vi "Create Config File Header.vi"(8 "error in (no error)":errorcluster, 11 "file path":path) -> (0 "error out":errorcluster, 3 "new file path":path)   [LabVIEW 2018, in "Config_Read_SPI.lvclass"]
uses:
  Config_Read_SPI.lvclass
  <vilib>/Utility/file.llb/Write Delimited Spreadsheet (string).vi
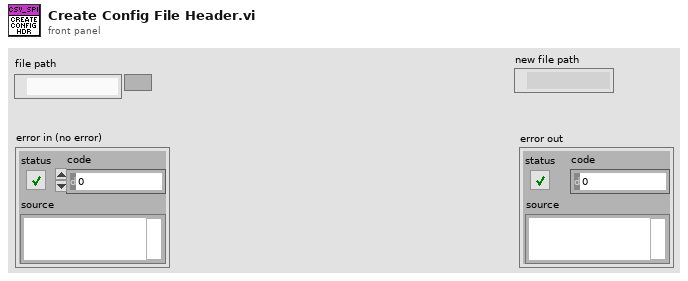
[diagram p1: front panel]
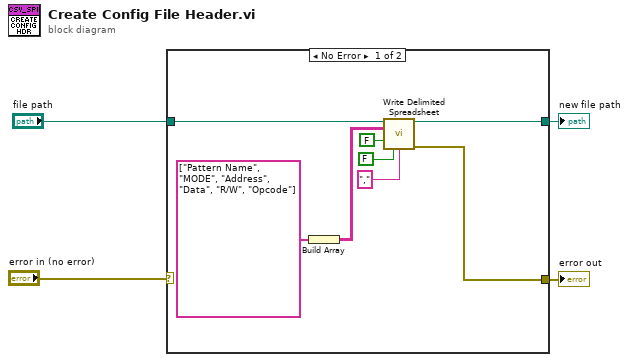
[diagram p0: block diagram]
diagram:
  n1 = case shown="No Error" "error in (no error)" {
    selector: "error in (no error)" -> [_ w13]
    tunnel: "file path" -> [w10 w14]
    tunnel: [w9 w13] -> w1
    tunnel: [w8 w14] -> w2
    frame No Error {
      n2 = Build Array(string[] ["Pattern Name", "MODE", "Address", "Data", "R/W", "Opcode"]) -> (w6:string[][])
      n3 = call-poly <vilib>:"Write Delimited Spreadsheet.vi"("file path (dialog if empty)"=w10, "2D data"=w6, "append to file? (new file:F)"=FALSE, "transpose? (no:F)"=FALSE, "delimiter (\\t)"="," ("delimiter (\\t)")) -> ("new file path (Not A Path if cancelled)"=w8:path, "error out"=w9:errorcluster)  [unwired: 9 in]
    }
    frame Error {
    }
  }
  "new file path" <- w2
  "error out" <- w1
